vi "Set XY Graph To Normal.vi"(9 "Cameras Number":i32, 11 "XY Graph Reference In":refnum<vi>) -> (3 "XY Graph Reference Out":refnum<vi>)   [LabVIEW 2022 SP3]
uses:
  Set XY Graph Line Color.vi
  Set XY Graph Point Color.vi
  Set XY Graph Interpolation Style.vi
  Set XY Graph Point Style.vi
  Set XY Graph Bar Style.vi
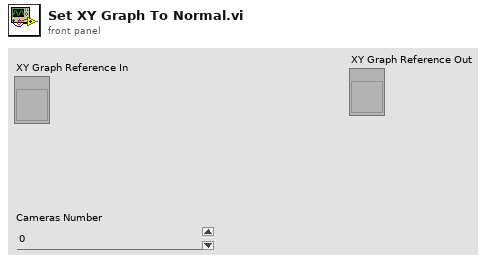
[diagram p1: front panel]
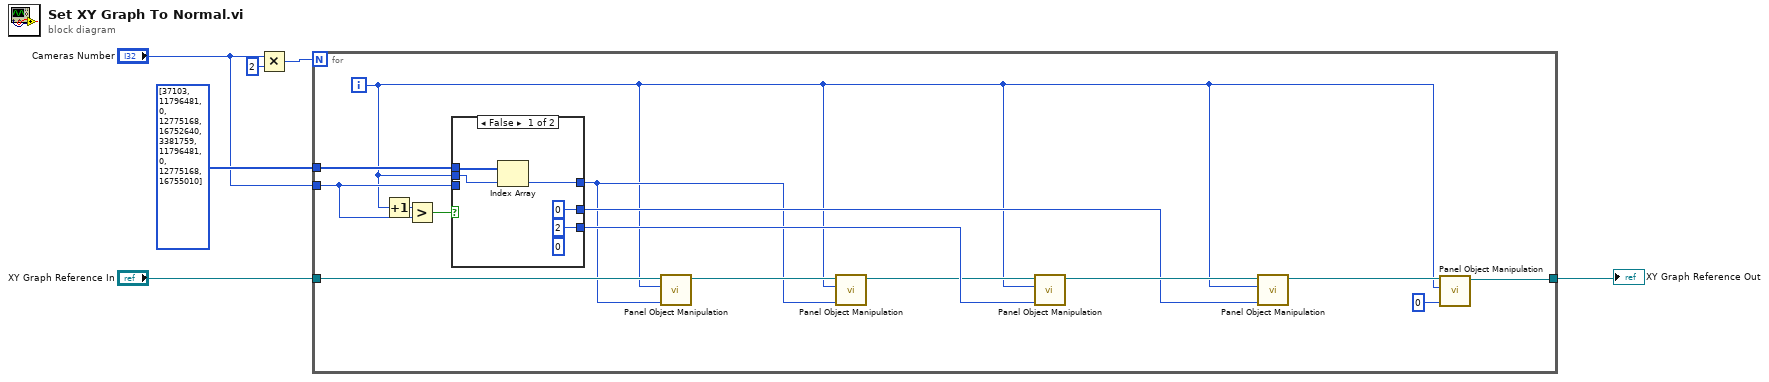
[diagram p0: block diagram]
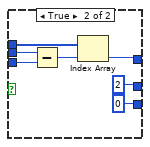
[diagram p2: hidden frame]
diagram:
  n1 = Multiply(x="Cameras Number", y=2) -> (x*y=w6:i32)
  n2 = for {
    N: w6 -> [_]
    tunnel: "XY Graph Reference In" -> [w19]
    tunnel: "Cameras Number" -> [w17]
    tunnel: [w13] -> w3
    tunnel: u32[] [37103, 11796481, 0, 12775168, 16752640, 3381759, 11796481, 0, 12775168, 16755010] -> [w18]
    i -> [w7]
    n3 = Increment(x=w7) -> (x+1=w11:i32)
    n4 = Greater?(x=w11, y=w17) -> (0:w21:bool)
    n5 = case shown="False" w21 {
      tunnel: w18 -> [w26 w33]
      tunnel: w17 -> [_ w32]
      tunnel: [w25 w29] -> w8
      tunnel: w7 -> [w22 w31]
      tunnel: [u8 2 ("Bar Style") u8 0 ("Bar Style")] -> w16
      tunnel: [u8 0 ("Point Style") u8 2 ("Point Style")] -> w15
      frame False {
        (unwired) u8 0 ("Bar Style")
        n6 = Index Array(array=w26, index=w22) -> (element=w25:u32)
      }
      frame True {
        n7 = Subtract(x=w31, y=w32) -> (x-y=w30:i32)
        n8 = Index Array(array=w33, index=w30) -> (element=w29:u32)
      }
    }
    n9 = call-poly "Panel Object Manipulation.vi"("Color"=w8, "Active Plot Start"=w7, "XY Graph Reference In"=w19) -> ("XY Graph Reference Out"=w10:refnum<vi>)  [unwired: 8 in]
    n10 = call-poly "Panel Object Manipulation.vi"("Point Color"=w8, "Active Plot Start"=w7, "XY Graph Reference In"=w10) -> ("XY Graph Reference Out"=w9:refnum<vi>)  [unwired: 8 in]
    n11 = call-poly "Panel Object Manipulation.vi"("InterPolation Style"=w16, "Active Plot Start"=w7, "XY Graph Reference In"=w9) -> ("XY Graph Reference Out"=w20:refnum<vi>)  [unwired: 8 in]
    n12 = call-poly "Panel Object Manipulation.vi"("Point Style"=w15, "Active Plot Start"=w7, "XY Graph Reference In"=w20) -> ("XY Graph Reference Out"=w14:refnum<vi>)  [unwired: 8 in]
    n13 = call-poly "Panel Object Manipulation.vi"("Bar Style"=u8 0, "Active Plot Start"=w7, "XY Graph Reference In"=w14) -> ("XY Graph Reference Out"=w13:refnum<vi>)  [unwired: 8 in]
  }
  "XY Graph Reference Out" <- w3
